vi "Set IPS Action Y.vi"(8 "error in (no error)":errorcluster, 10 "PSU Act Stat":T1="HOLD" caption="PSU Action Status", 11 "Instrument.OxfordVRM in":refnum<class "Instrument.OxfordVRM.lvclass">) -> (0 "error out":errorcluster, 2 "Response":string, 3 "Instrument.OxfordVRM out":refnum<class "Instrument.OxfordVRM.lvclass">)   [LabVIEW 2016, in "Instrument.OxfordVRM.lvclass"]
uses:
  Instrument.OxfordVRM.lvclass
  <instrlib>/Mercury iXX/Public/Libraries/Magnet/Controls/PSU Actions.ctl
  Instrument.OxfordVRM.lvclass/Instrument.OxfordVRM.ctl
  <instrlib>/Mercury iXX/Public/Libraries/Magnet/Open/Open Magnet Device.vi
  <instrlib>/Mercury iXX/Public/Libraries/Magnet/Configuration/Set/PSU Action Status (Set).vi
  <instrlib>/Mercury iXX/Public/Libraries/Magnet/Configuration/Read/PSU Action Status (Read).vi
  <instrlib>/Mercury iXX/Mercury iXX.lvlib
  <instrlib>/Mercury iXX/Public/Libraries/Magnet.lvlib
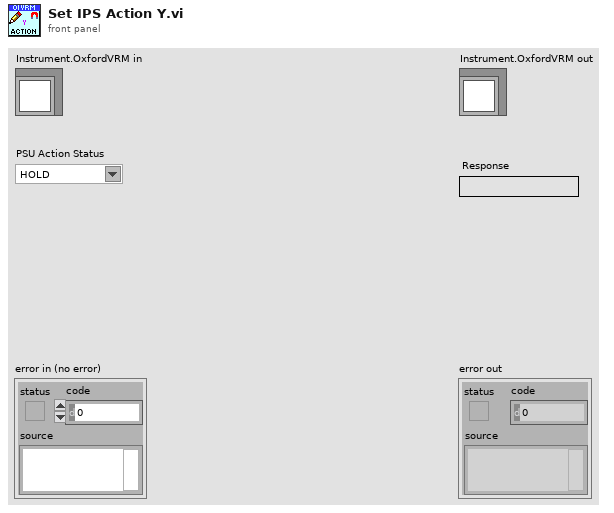
[diagram p1: front panel]
types:
  T1 = typedef "Mercury iXX.lvlib/Magnet.lvlib/PSU Actions.ctl" = string
  T2 = typedef "Mercury iXX.lvlib/Mercury Reference.ctl" = cluster{"Comms":refnum<visa-resource-name>, "Device ID":string[], "Comms Layer":T3, "Command":string, "Query reference":T4}
  T3 = typedef "Mercury iXX.lvlib/Comms Transport Layer.ctl" = enum16{"Ethernet TCP/IP", "USB", "ISOBus - RS-232", "GPIB"}
  T4 = typedef "Mercury iXX.lvlib/Query Dynamic Reference.ctl" = refnum<vi>
  T5 = typedef "Mercury iXX.lvlib/Response String.ctl" = string
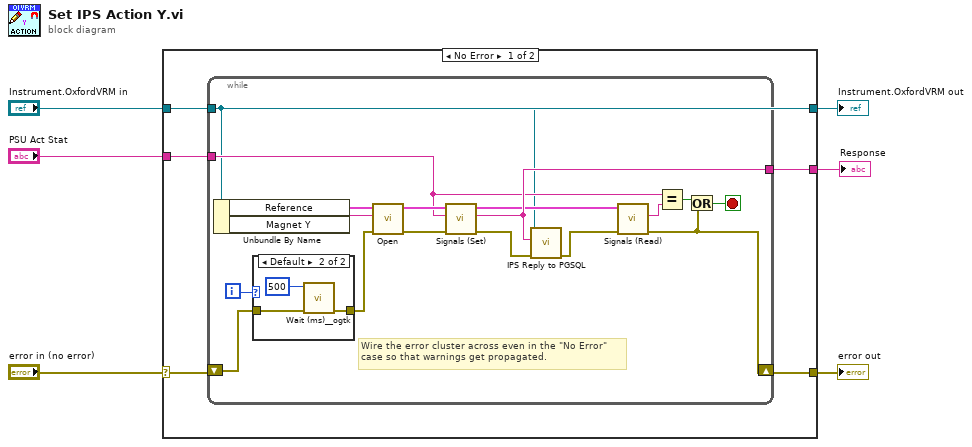
[diagram p0: block diagram]
diagram:
  n1 = case shown="No Error" "error in (no error)" {
    selector: "error in (no error)" -> [w10 w34]
    tunnel: [w8 w34] -> w5
    tunnel: [w11 w33] -> w3
    tunnel: "Instrument.OxfordVRM in" -> [w11 w33]
    tunnel: [w9 _] -> w2
    tunnel: "PSU Act Stat" -> [w7 _]
    frame No Error {
      n2 = while {
        tunnel: w11 -> [w15]
        tunnel: [w23] -> w9
        tunnel: w7 -> [w21]
        shift-right: [w14] -> w8
        shift-left: w10 -> [w18]
        i -> [w17]
        stop <- w12 stop-if-true
        # "Wire the error cluster across even in the \"No Error\"\ncase so that warnings get propagated."
        n3 = Unbundle By Name(w15) -> ("Reference"=w27:T2, "Magnet Y"=w28:string)
        n4 = case shown="Default" w17 {
          tunnel: w18 -> [w29 w32]
          tunnel: [w29 w31] -> w16
          frame 0 {
          }
          frame Default {
            n5 = call <userlib>:"Wait (ms)__ogtk.vi"("error in (no error)"=w32, "milliseconds to wait"=u32 500) -> ("error out"=w31:errorcluster)  [unwired: 8 in, 1 out]
          }
        }
        n6 = call-poly <instrlib>:"Open.vi"("error in (no error)"=w16, "Device Identifier"=w28, "Mercury Reference In"=w27) -> ("error out"=w25:errorcluster, "Mercury Reference Out"=w26:T2)  [unwired: 7 out]
        n7 = call-poly <instrlib>:"Signals (Set).vi"("error in"=w25, "PSU Act Stat"=w21, "Mercury Reference In"=w26) -> ("error out"=w24:errorcluster, "Response"=w23:T5, "Mercury Reference Out"=w22:T2)  [unwired: 1 in, 5 out]
        n8 = call "IPS Reply to PGSQL.vi"("error in (no error)"=w24, "Response"=w23, "Instrument.1820 in"=w15) -> ("error out"=w20:errorcluster)  [unwired: 7 in, 1 out]
        n9 = call-poly <instrlib>:"Signals (Read).vi"("error in"=w20, "Mercury Reference In"=w22) -> ("error out"=w14:errorcluster, "PSU Act Stat"=w19:T1)  [unwired: 1 in, 7 out]
        n10 = Equal?(x=w21, y=w19) -> (x = y?=w13:bool)
        n11 = Or(x=w13, y=w14) -> (x .or. y?=w12:bool)
      }
    }
    frame Error {
    }
  }
  "error out" <- w5
  "Instrument.OxfordVRM out" <- w3
  "Response" <- w2
